vi "UART_With_Buffer.vi"(0 "COM":refnum<visa-resource-name>, 1 "Timeout (ms)":u32=500, 5 "Function":T1(ring)=enum."SendWaitRead", 7 "Send":string(combo), 9 "Baudrate":u32=115200, 11 "error in (no error)":errorcluster, 12 "Read regular":string="\n") -> (4 "ReceiveString":string, 15 "error out":errorcluster)   [LabVIEW 2020]
uses:
  <vilib>/Instr/_visa.llb/VISA Set IO Buffer Mask.ctl
  <vilib>/Instr/_visa.llb/VISA Flush IO Buffer Mask.ctl
  <vilib>/Instr/_visa.llb/VISA Configure Serial Port (Instr).vi
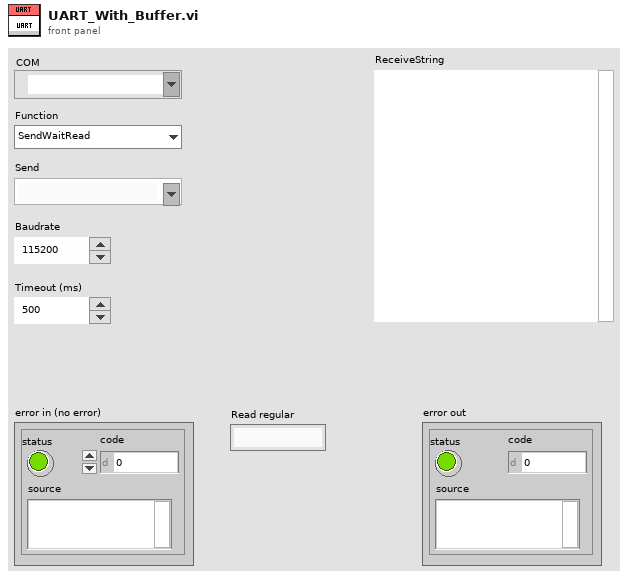
[diagram p1: front panel]
types:
  T1 = enum16{"Open", "Close", "ClearBuffer", "Send", "Read", "SendWaitRead"}
  T2 = enum16{"Open", "Close", "ClearBuffer", "Send", "Read", "SendWaitRead", "SendCompare", "ReadCompare"}
  T3 = typedef "VISA Set IO Buffer Mask.ctl" = u16
  T4 = typedef "VISA Flush IO Buffer Mask.ctl" = u16
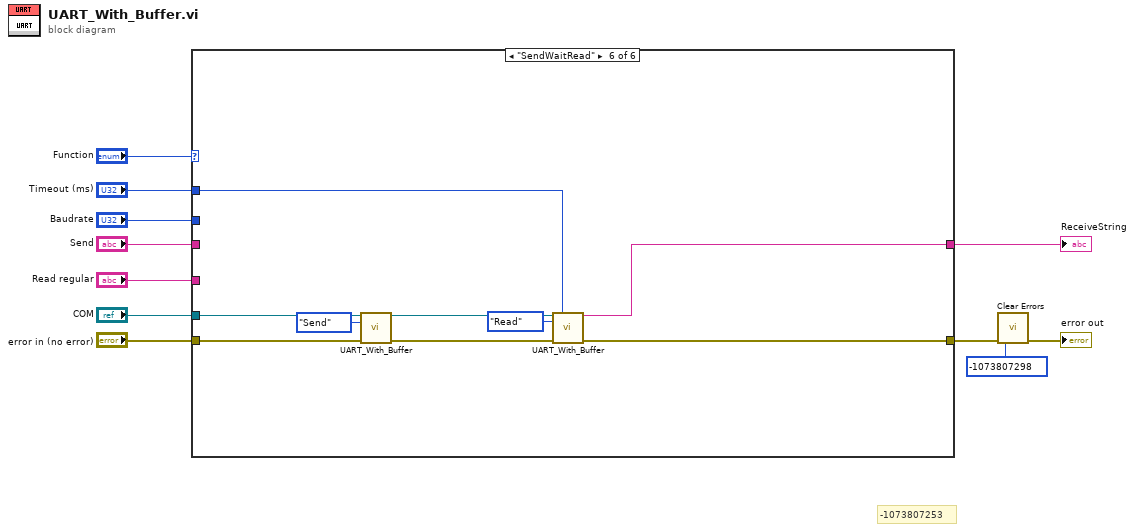
[diagram p0: block diagram]
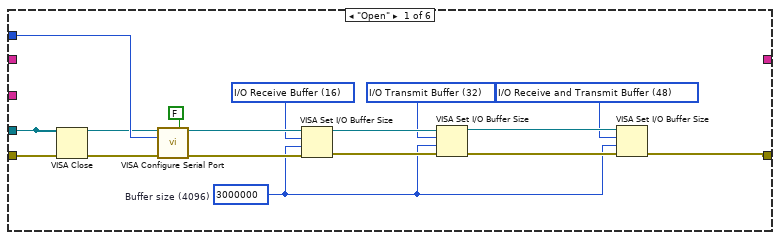
[diagram p2: hidden frame]
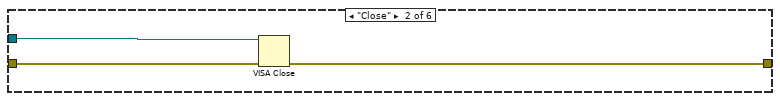
[diagram p3: hidden frame]
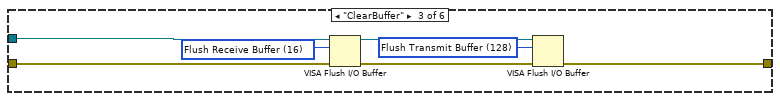
[diagram p4: hidden frame]
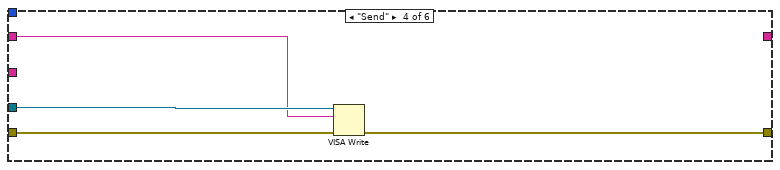
[diagram p5: hidden frame]
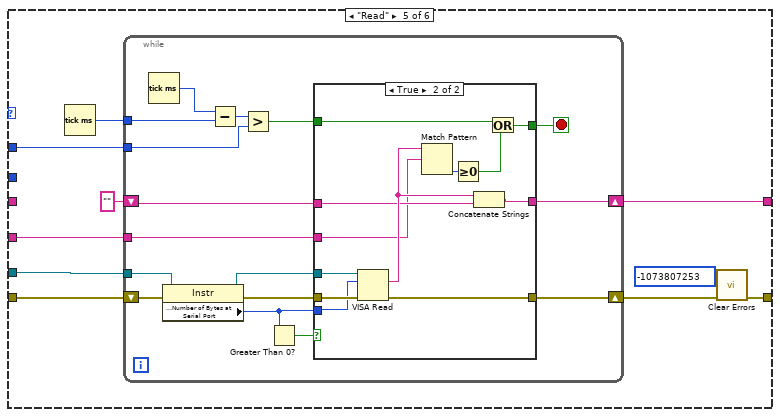
[diagram p6: hidden frame]
diagram:
  # "-1073807253"
  n1 = case shown="\"SendWaitRead\"" "Function" {
    tunnel: "Send" -> [_ _ _ w38 _ _]
    tunnel: "error in (no error)" -> [w24 w29 w33 w40 w50 w86]
    tunnel: [w12 w28 w36 w41 w46 w89] -> w4
    tunnel: "COM" -> [w25 w30 w32 w39 w51 w87]
    tunnel: "Baudrate" -> [w27 _ _ _ _ _]
    tunnel: "Timeout (ms)" -> [_ _ _ _ w45 w82]
    tunnel: [_ _ _ _ w49 w85] -> w2
    tunnel: "Read regular" -> [_ _ _ _ w42 _]
    frame "Open" {
      w13 = T3 16 items=["I/O Receive Buffer"=16, "I/O Transmit Buffer"=32, "I/O Receive and Transmit Buffer"=48] ("Mask")
      w14 = T3 48 items=["I/O Receive Buffer"=16, "I/O Transmit Buffer"=32, "I/O Receive and Transmit Buffer"=48] ("Mask")
      w15 = T3 32 items=["I/O Receive Buffer"=16, "I/O Transmit Buffer"=32, "I/O Receive and Transmit Buffer"=48] ("Mask")
      w16 = u32 3000000  # Buffer size (4096)
      n2 = VISA Close(VISA resource name=w25, error in (no error)=w24) -> (error out=w23:errorcluster)
      n3 = call-poly "VISA Configure Serial Port"("VISA resource name"=w25, "Enable Termination\nChar (T)"=FALSE ("Enable Termination\nChar (T)"), "baud rate (9600)"=w27, "error in (no error)"=w23) -> ("VISA resource name out"=w21:refnum<visa-resource-name>, "error out"=w22:errorcluster)  [unwired: 4 in, 6 out]
      n4 = VISA Set I/O Buffer Size(VISA resource name=w21, mask (16)=w13, size (4096)=w16, error in (no error)=w22) -> (VISA resource name out=w20:refnum<visa-resource-name>, error out=w18:errorcluster)
      n5 = VISA Set I/O Buffer Size(VISA resource name=w20, mask (16)=w15, size (4096)=w16, error in (no error)=w18) -> (VISA resource name out=w19:refnum<visa-resource-name>, error out=w17:errorcluster)
      n6 = VISA Set I/O Buffer Size(VISA resource name=w19, mask (16)=w14, size (4096)=w16, error in (no error)=w17) -> (error out=w12:errorcluster)  [unwired: 1 out]
    }
    frame "Close" {
      n7 = VISA Close(VISA resource name=w30, error in (no error)=w29) -> (error out=w28:errorcluster)
    }
    frame "ClearBuffer" {
      w35 = T4 16 items=["Flush Receive Buffer"=16, "Write Transmit Buffer to Device"=32, "Flush Receive Buffer (No I/O)"=64, "Flush Transmit Buffer"=128] ("Mask")
      w37 = T4 128 items=["Flush Receive Buffer"=16, "Write Transmit Buffer to Device"=32, "Flush Receive Buffer (No I/O)"=64, "Flush Transmit Buffer"=128] ("Mask")
      n8 = VISA Flush I/O Buffer(VISA resource name=w32, mask (16)=w35, error in (no error)=w33) -> (VISA resource name out=w31:refnum<visa-resource-name>, error out=w34:errorcluster)
      n9 = VISA Flush I/O Buffer(VISA resource name=w31, mask (16)=w37, error in (no error)=w34) -> (error out=w36:errorcluster)  [unwired: 1 out]
    }
    frame "Send" {
      n10 = VISA Write(VISA resource name=w39, write buffer=w38, error in (no error)=w40) -> (error out=w41:errorcluster)  [unwired: 2 out]
    }
    frame "Read" {
      n11 = Tick Count (ms)() -> (millisecond timer value=w44:u32)
      n12 = while {
        tunnel: w51 -> [w67]
        shift-right: [w62] -> w47
        shift-left: w50 -> [w54]
        tunnel: w45 -> [w57]
        tunnel: w44 -> [w59]
        shift-right: [w63] -> w49
        shift-left: "" ("read buffer") -> [w55]
        tunnel: w42 -> [w52]
        stop <- w61 stop-if-true
        n13 = Tick Count (ms)() -> (millisecond timer value=w60:u32)
        n14 = property class="Instr"(reference=w67, error in=w54) -> (reference out=w66:refnum<visa-resource-name>, error out=w53:errorcluster, "Serial Settings:Number of Bytes at Serial Port"=w65:u32)
        n15 = Subtract(x=w60, y=w59) -> (x-y=w58:u32)
        n16 = Greater?(x=w58, y=w57) -> (0:w56:bool)
        n17 = Greater Than 0?(x=w65) -> (x > 0?=w64:bool)
        n18 = case shown="True" w64 {
          tunnel: [w69 w81] -> w62
          tunnel: w53 -> [w69 w80]
          tunnel: w66 -> [_ w79]
          tunnel: [_ w73] -> w63
          tunnel: w65 -> [_ w71]
          tunnel: [w68 w76] -> w61
          tunnel: w56 -> [w68 w74]
          tunnel: w55 -> [_ w72]
          tunnel: w52 -> [_ w70]
          frame False {
          }
          frame True {
            n19 = VISA Read(VISA resource name=w79, byte count=w71, error in (no error)=w80) -> (read buffer=w78:string, error out=w81:errorcluster)  [unwired: 2 out]
            n20 = Match Pattern(string=w78, regular expression=w70) -> (offset past match=w77:i32)  [unwired: 1 in, 3 out]
            n21 = Greater Or Equal To 0?(x=w77) -> (x >= 0?=w75:bool)
            n22 = Concatenate Strings(w78, w72) -> (w73:string)
            n23 = Or(x=w74, y=w75) -> (x .or. y?=w76:bool)
          }
        }
      }
      n24 = call <vilib>:"Clear Errors.vi"("error in (no error)"=w47, "specific error code to clear (0: all)"=-1073807253) -> ("error out"=w46:errorcluster)  [unwired: 4 in, 1 out]
    }
    frame "SendWaitRead" {
      n25 = call "UART_With_Buffer.vi"("COM"=w87, "Function"=T2."Send", "error in (no error)"=w86) -> ("error out"=w88:errorcluster)  [unwired: 11 in, 1 out]
      n26 = call "UART_With_Buffer.vi"("COM"=w87, "Timeout (ms)"=w82, "Function"=T2."Read", "error in (no error)"=w88) -> ("ReceiveString"=w85:string, "error out"=w89:errorcluster)  [unwired: 10 in]
    }
  }
  "ReceiveString" <- w2
  n27 = call <vilib>:"Clear Errors.vi"("error in (no error)"=w4, "specific error code to clear (0: all)"=-1073807298) -> ("error out"=→"error out":errorcluster)  [unwired: 4 in, 1 out]
